vi "Main.vi"() -> ()   [LabVIEW 2009]
uses:
  Action Engines/AE Cores/Custom Controls/WiimoteState.ctl
  Action Engines/AE Access VIs/AE - Bluetooth Get Reference.vi
  Action Engines/AE Access VIs/AE - Bluetooth Battery.vi
  Action Engines/AE Access VIs/AE - Bluetooth ButtonAccData.vi
  Action Engines/AE Access VIs/AE - Bluetooth Connect All.vi
  Action Engines/AE Access VIs/AE - Bluetooth Initialise.vi
  Action Engines/AE Access VIs/AE - Bluetooth Pair All.vi
panel:
  out "Battery Raw":u8
  out "Battery Level":dbl
  out "Wiimote State":T1
  in  "Volume":u8=255 format="%x"
  in  "stop":bool
  in  "Number of retries":i32=3
  in  "No. of Wiimotes":i32=1
  out "No. of Wiimotes Paired":i32
  in  "error in (no error)":errorcluster
  # "Accelerometers"
  # "Buttons"
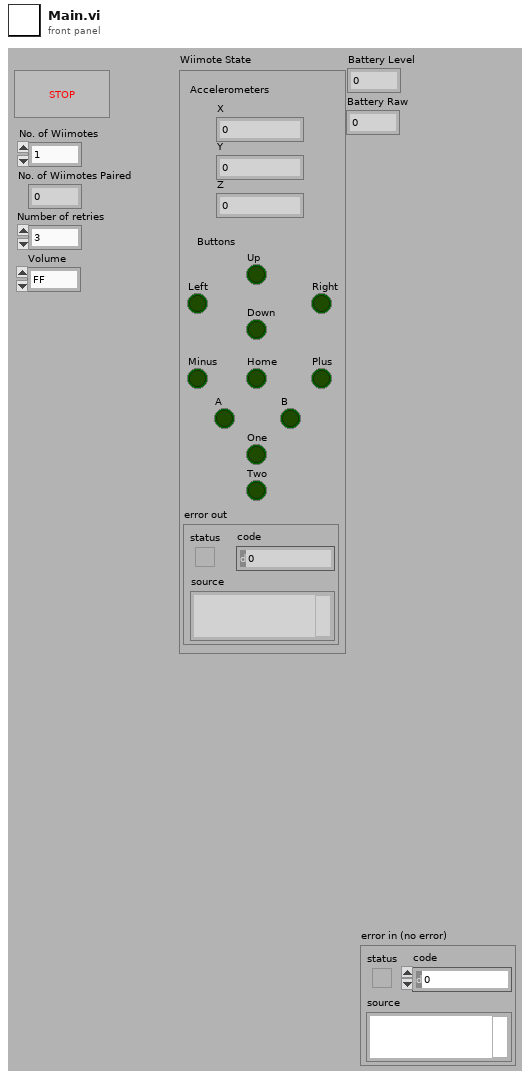
[diagram p1: front panel]
types:
  T1 = typedef "WiimoteState.ctl" = cluster{"X":sgl, "Y":sgl, "Z":sgl, "A":bool, "B":bool, "Down":bool, "Home":bool, "Left":bool, "Minus":bool, "One":bool, "Plus":bool, "Right":bool, "Two":bool, "Up":bool, "error out":errorcluster}
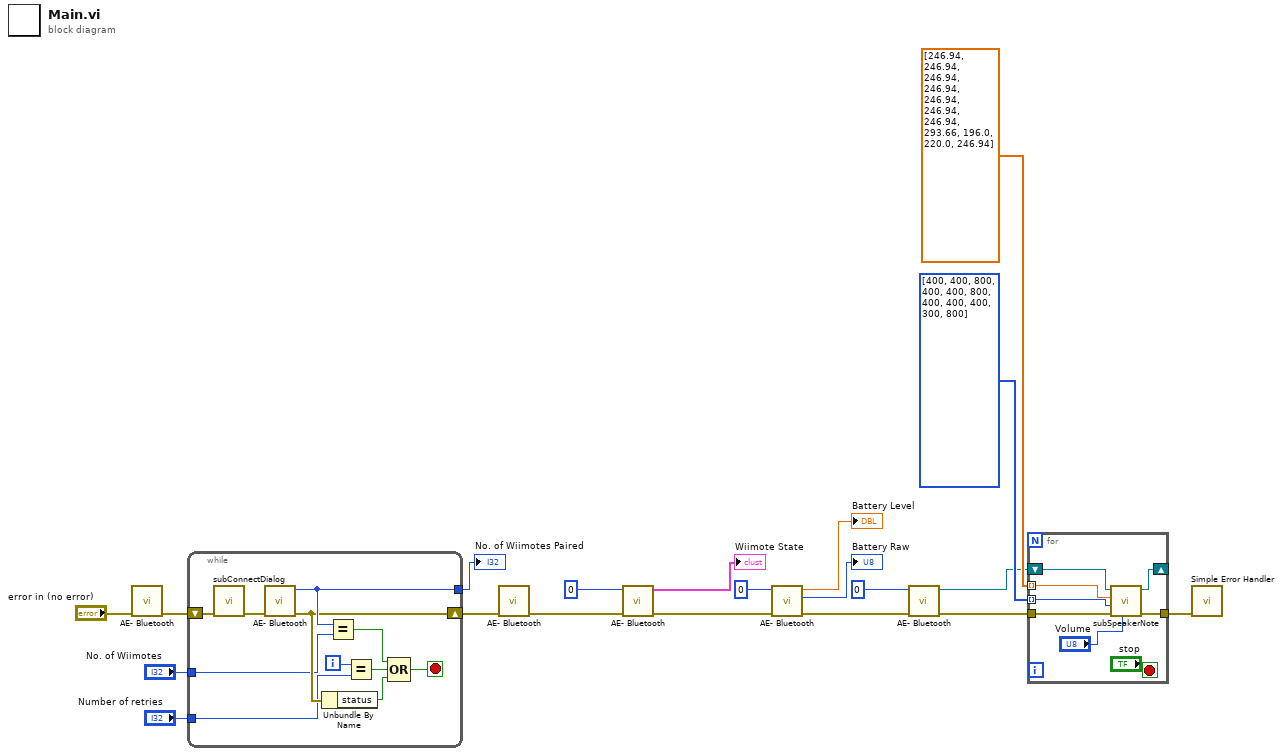
[diagram p0: block diagram]
diagram:
  w13 = dbl[] [246.94, 246.94, 246.94, 246.94, 246.94, 246.94, 246.94, 293.66, 196.0, 220.0, 246.94] items=["D3"=146.83, "E3"=164.81, "F3"=174.61, "G3"=196.0, "A3"=220.0, "B3"=246.94, "C4"=261.63, "D4"=293.66, "E4"=329.63, "F4"=349.23, "G4"=392.0, "A4"=440.0]
  n1 = call-poly "AE- Bluetooth.vi"("error in (no error)"="error in (no error)") -> ("error out"=w19:errorcluster)  [unwired: 10 in]
  n2 = while {
    tunnel: [w25] -> w18
    shift-right: [w24] -> w20
    shift-left: w19 -> [w27]
    tunnel: "No. of Wiimotes" -> [w22]
    tunnel: "Number of retries" -> [w21]
    i -> [w30]
    stop <- w28 stop-if-true
    n3 = call "subConnectDialog.vi"("error in (no error)"=w27) -> ("error out"=w26:errorcluster)  [unwired: 10 in]
    n4 = call-poly "AE- Bluetooth.vi"("error in (no error)"=w26) -> ("error out"=w24:errorcluster, "Number of wiimotes paired"=w25:i32)  [unwired: 9 in]
    n5 = Unbundle By Name(w24) -> ("status"=w23:bool)
    n6 = Equal?(x=w25, y=w22) -> (x = y?=w31:bool)
    n7 = Equal?(x=w30, y=w21) -> (x = y?=w29:bool)
    n8 = Compound Arithmetic op=OR(w31, w29, w23) -> (w28:bool)
  }
  "No. of Wiimotes Paired" <- w18
  n9 = call-poly "AE- Bluetooth.vi"("error in (no error)"=w20) -> ("error out"=w9:errorcluster)  [unwired: 9 in, 1 out]
  n10 = call-poly "AE- Bluetooth.vi"("error in (no error)"=w9, "Wiimote"=0) -> ("error out"=w7:errorcluster, "Wiimote State"=→"Wiimote State":T1)  [unwired: 8 in]
  n11 = call-poly "AE- Bluetooth.vi"("error in (no error)"=w7, "Wiimote"=u8 0) -> ("error out"=w6:errorcluster, "Battery Raw"=→"Battery Raw":u8, "Battery Level"=→"Battery Level":dbl)  [unwired: 7 in]
  n12 = call-poly "AE- Bluetooth.vi"("error in (no error)"=w6, "Wiimote"=u8 0) -> ("error out"=w11:errorcluster, "Wiimote Reference"=w10:refnum<k24>)  [unwired: 8 in]
  n13 = for {
    tunnel: [w37] -> w14
    tunnel: w11 -> [w39]
    tunnel: w13 -> [w36] mode=indexing
    shift-right: [w33] -> _
    shift-left: w10 -> [w34]
    tunnel: i32[] [400, 400, 800, 400, 400, 800, 400, 400, 400, 300, 800] -> [w32] mode=indexing
    stop <- "stop" stop-if-true
    n14 = call "subSpeakerNote.vi"("Volume"="Volume", "error in"=w39, "Note Duration (ms)"=w32, "Desired Freq"=w36, "reference"=w34) -> ("error out"=w37:errorcluster, "reference out"=w33:refnum<k24>)  [unwired: 5 in]
  }
  n15 = call <vilib>:"Simple Error Handler.vi"("error in (no error)"=w14) -> ()  [unwired: 4 in, 5 out]
